vi "Error Query.vi"(0 "VISA resource name":refnum<visa-resource-name>, 11 "error in (no error)":errorcluster) -> (4 "VISA resource name out":refnum<visa-resource-name>, 6 "Error Code":i32, 8 "Error Message":string, 15 "error out":errorcluster)   [LabVIEW 2014, in "Associated Power Technologies 8500 Series.lvlib"]
doc: "Queries the instrument for any errors in the instrument's error queue. It will continue to read errors until all errors have been read from the instrument. Any errors will be returned in the <B>error out</B> control.\n\n<B>Note:</B>\nThis VI is called automatically by most driver VIs so it is not usually necessary to call this in an application."
uses:
  <instrlib>/Associated Power Technologies 8500 Series/Associated Power Technologies 8500 Series.lvlib
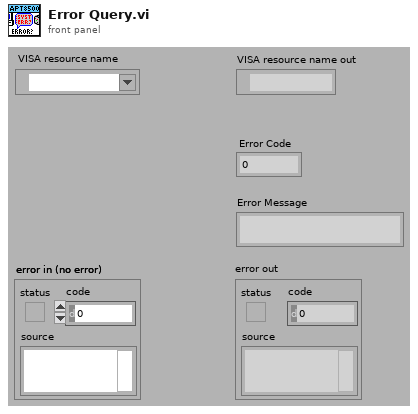
[diagram p1: front panel]
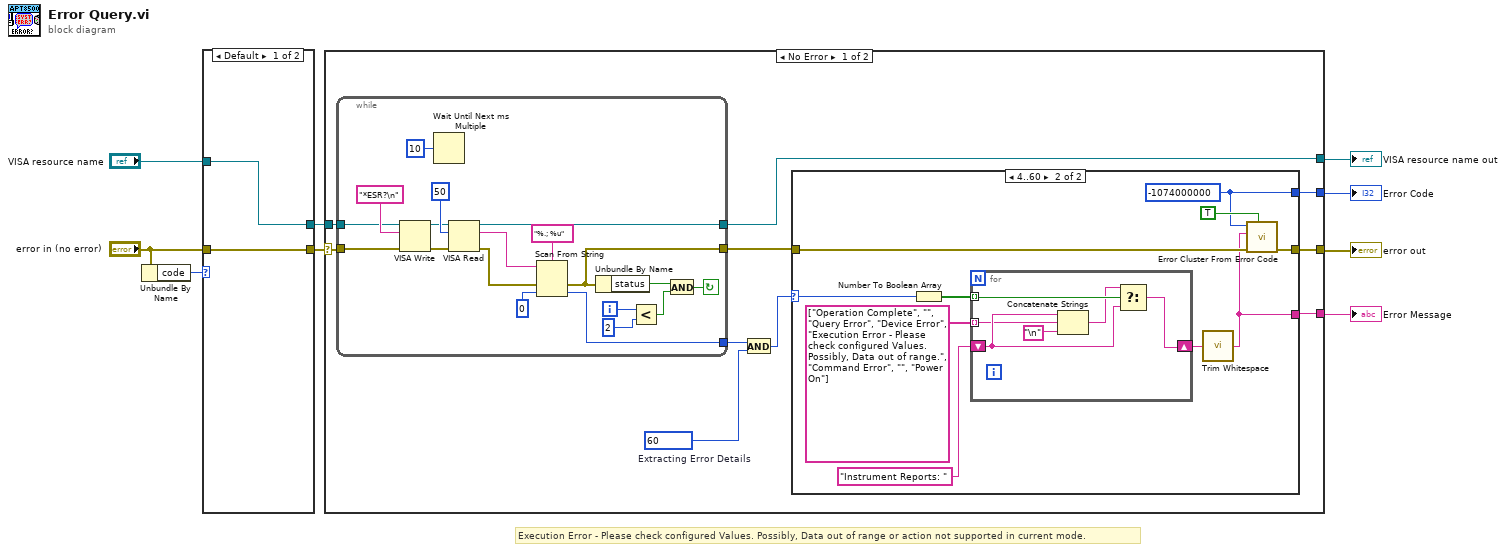
[diagram p0: block diagram]
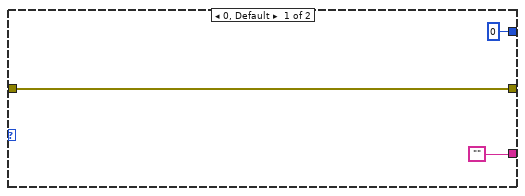
[diagram p2: hidden frame]
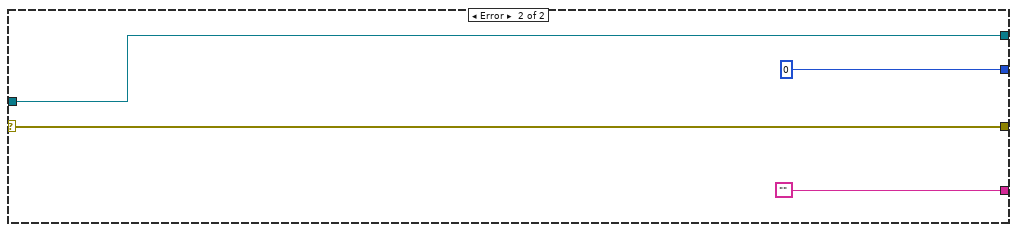
[diagram p3: hidden frame]
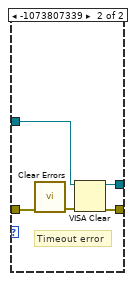
[diagram p4: hidden frame]
diagram:
  # "Execution Error - Please check configured Values. Possibly, Data out of range or action not supported in current mode."
  n1 = Unbundle By Name("error in (no error)") -> ("code"=w3:i32)
  n2 = case shown="Default" w3 {
    tunnel: "error in (no error)" -> [w11 w16]
    tunnel: "VISA resource name" -> [w10 w14]
    tunnel: [w11 w12] -> w4
    tunnel: [w10 w15] -> w5
    frame Default {
    }
    frame -1073807339 {
      # "Timeout error"
      n3 = call <vilib>:"Clear Errors.vi"("error in (no error)"=w16) -> ("error out"=w13:errorcluster)  [unwired: 5 in, 1 out]
      n4 = VISA Clear(VISA resource name=w14, error in (no error)=w13) -> (VISA resource name out=w15:refnum<visa-resource-name>, error out=w12:errorcluster)
    }
  }
  n5 = case shown="No Error" w4 {
    selector: w4 -> [w20 w68]
    tunnel: [w17 w67] -> w9
    tunnel: [w26 w68] -> w8
    tunnel: w5 -> [w21 w67]
    tunnel: [w23 "" ("Empty String Constant")] -> w2
    tunnel: [w22 0 ("Code")] -> w1
    frame No Error {
      w25 = u8 60  # Extracting Error Details
      n6 = while {
        tunnel: [w29] -> w17
        tunnel: w20 -> [w34]
        tunnel: w21 -> [w30]
        tunnel: [w28] -> w19
        tunnel: [w27] -> w18
        i -> [w40]
        stop <- w36 continue-if-true
        n7 = VISA Write(VISA resource name=w30, write buffer="*ESR?\n" ("Command to Send (empty)"), error in (no error)=w34) -> (VISA resource name out=w32:refnum<visa-resource-name>, error out=w33:errorcluster)  [unwired: 1 out]
        n8 = Wait Until Next ms Multiple(millisecond multiple=u32 10) -> ()  [unwired: 1 out]
        n9 = VISA Read(VISA resource name=w32, byte count=u32 50, error in (no error)=w33) -> (VISA resource name out=w29:refnum<visa-resource-name>, read buffer=w44:string, error out=w41:errorcluster)  [unwired: 1 out]
        n10 = Scan From String(format string="%.; %u" ("Format String"), input string=w44, error in=w41, default 1=u8 0 ("default value 1")) -> (error out=w27:errorcluster, output 1=w28:u8)  [unwired: 1 in, 2 out]
        n11 = Unbundle By Name(w27) -> ("status"=w37:bool)
        n12 = Less?(x=w40, y=2) -> (x < y?=w38:bool)
        n13 = And(x=w37, y=w38) -> (x .and. y?=w36:bool)
      }
      n14 = And(x=w19, y=w25) -> (x .and. y?=w24:u8)
      n15 = case shown="4..60" w24 {
        selector: w24 -> [_ w52]
        tunnel: [w48 w51] -> w26
        tunnel: w18 -> [w48 w55]
        tunnel: ["" ("Empty String Constant") w50] -> w23
        tunnel: [0 ("Code") w49] -> w22
        frame 0, Default {
        }
        frame 4..60 {
          w49 = -1074000000 ("Code")
          n16 = Number To Boolean Array(number=w52) -> (Boolean array=w57:bool[])
          n17 = for {
            tunnel: w57 -> [w64] mode=indexing
            tunnel: string[] ["Operation Complete", "", "Query Error", "Device Error", "Execution Error - Please check configured Values. Possibly, Data out of range.", "Command Error", "", "Power On"] -> [w61] mode=indexing
            shift-right: [w63] -> w54
            shift-left: "Instrument Reports: " -> [w62]
            n18 = Concatenate Strings(w62, w61, "\n" ("Line Feed Constant")) -> (w60:string)
            n19 = Select(t=w60, s=w64, f=w62) -> (s? t:f=w63:string)
          }
          n20 = call <vilib>:"Trim Whitespace.vi"("string"=w54) -> ("trimmed string"=w50:string)  [unwired: 1 in]
          n21 = call <vilib>:"Error Cluster From Error Code.vi"("show call chain? (False)"=TRUE, "error in (no error)"=w55, "error message (\"\")"=w50, "error code (0)"=w49) -> ("error out"=w51:errorcluster)  [unwired: 5 in]
        }
      }
    }
    frame Error {
    }
  }
  "VISA resource name out" <- w9
  "error out" <- w8
  "Error Message" <- w2
  "Error Code" <- w1
